vi "ctrl string.vi"(11 "read buffer":string) -> (0 "nCannone":i32, 2 "vel":i32, 3 "angolo":i32)   [LabVIEW 2017]
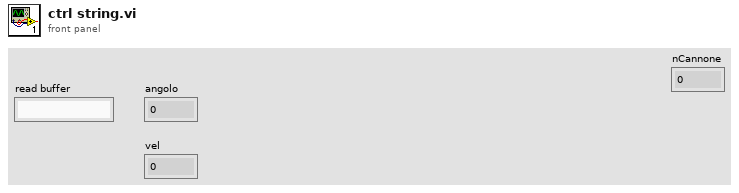
[diagram p1: front panel]
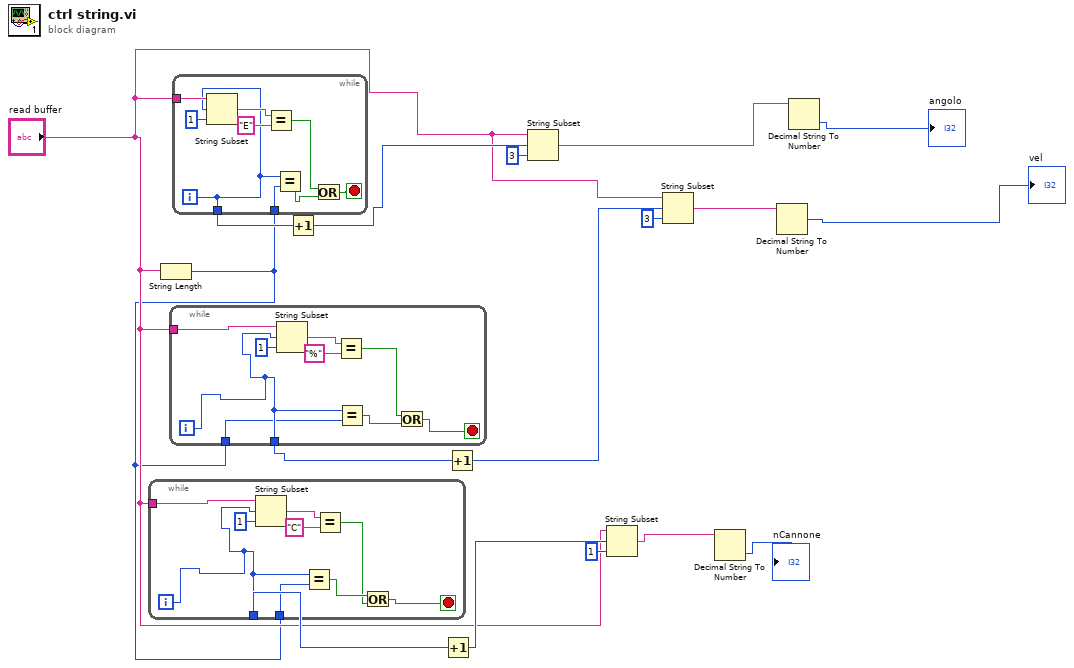
[diagram p0: block diagram]
diagram:
  n1 = String Length(string="read buffer") -> (length=w1:i32)
  n2 = while {
    tunnel: "read buffer" -> [w26]
    tunnel: [w22] -> w7
    tunnel: w1 -> [w20]
    i -> [w22]
    stop <- w18 stop-if-true
    n3 = String Subset(string=w26, offset (0)=w22, length (rest)=1 ("length (rest)")) -> (substring=w25:string)
    n4 = Equal?(x=w22, y=w20) -> (x = y?=w21:bool)
    n5 = Equal?(x=w25, y="C") -> (x = y?=w19:bool)
    n6 = Or(x=w21, y=w19) -> (x .or. y?=w18:bool)
  }
  n7 = while {
    tunnel: "read buffer" -> [w35]
    tunnel: [w28] -> w11
    tunnel: w1 -> [w27]
    i -> [w28]
    stop <- w31 stop-if-true
    n8 = String Subset(string=w35, offset (0)=w28, length (rest)=1 ("length (rest)")) -> (substring=w34:string)
    n9 = Equal?(x=w34, y="%") -> (x = y?=w30:bool)
    n10 = Equal?(x=w28, y=w27) -> (x = y?=w29:bool)
    n11 = Or(x=w30, y=w29) -> (x .or. y?=w31:bool)
  }
  n12 = while {
    tunnel: "read buffer" -> [w44]
    tunnel: [w39] -> w13
    tunnel: w1 -> [w38]
    i -> [w39]
    stop <- w37 stop-if-true
    n13 = String Subset(string=w44, offset (0)=w39, length (rest)=1 ("length (rest)")) -> (substring=w43:string)
    n14 = Equal?(x=w43, y="E") -> (x = y?=w41:bool)
    n15 = Equal?(x=w39, y=w38) -> (x = y?=w36:bool)
    n16 = Or(x=w41, y=w36) -> (x .or. y?=w37:bool)
  }
  n17 = Increment(x=w13) -> (x+1=w9:i32)
  n18 = Increment(x=w7) -> (x+1=w6:i32)
  n19 = Increment(x=w11) -> (x+1=w8:i32)
  n20 = String Subset(string="read buffer", offset (0)=w9, length (rest)=3 ("length (rest)")) -> (substring=w15:string)
  n21 = String Subset(string="read buffer", offset (0)=w6, length (rest)=1 ("length (rest)")) -> (substring=w4:string)
  n22 = String Subset(string="read buffer", offset (0)=w8, length (rest)=3 ("length (rest)")) -> (substring=w16:string)
  n23 = Decimal String To Number(string=w4) -> (number=→"nCannone":i32)  [unwired: 2 in, 1 out]
  n24 = Decimal String To Number(string=w16) -> (number=→"vel":i32)  [unwired: 2 in, 1 out]
  n25 = Decimal String To Number(string=w15) -> (number=→"angolo":i32)  [unwired: 2 in, 1 out]
